vi "empty task properties test.vi"() -> ()   [LabVIEW 2013]
uses:
  <resource>/objmgr/daqmx.rc
panel:
  out "error out":errorcluster
  out "Done":bool
  out "NumChans":u32
  out "Name":refnum<k21>
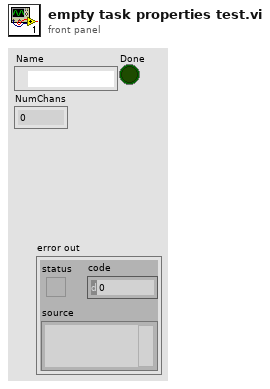
[diagram p1: front panel]
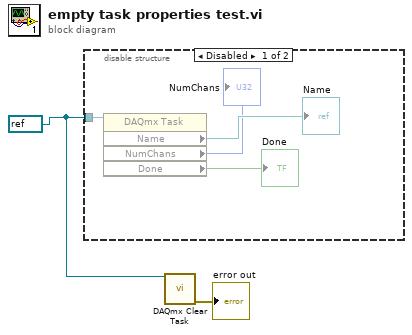
[diagram p0: block diagram]
diagram:
  w2 = refnum<k21> refnum ("y")
  n1 = disable-structure shown="Disabled" {
    disable-tunnel: w2 -> [w6 _]
    frame Disabled {
      n2 = property class="DAQmx Task"(reference=w6) -> ("Name"=→"Name":refnum<k21>, "NumChans"=→"NumChans":u32, "Done"=→"Done":bool)  [unwired: 1 in, 2 out]
    }
    frame Enabled {
    }
  }
  n3 = call <vilib>:"DAQmx Clear Task.vi"("task in"=w2) -> ("error out"=→"error out":errorcluster)  [unwired: 14 in]
